vi "NotifyRegistered.vi"(2 "data string":string, 3 "ROS":T1={"topic port"=0, "Node"="", "topic"="", "type"="", "node port"=0, "error "={"status"=FALSE, "code"=0, "source"=""}, "Direction"=enum."Node", "APIs"=[], "Update (ms)"=1, "write queue"=1}) -> (1 "ROS out":T1={"topic port"=0, "Node"="", "topic"="", "type"="", "node port"=0, "error "={"status"=FALSE, "code"=0, "source"=""}, "Direction"=enum."Node", "APIs"=[], "Update (ms)"=1, "write queue"=1})   [LabVIEW 2012]
uses:
  <userlib>/ROSforLV/ROS/Code/SubVIs/_ROSControl.ctl
  <userlib>/ROSforLV/ROS/Code/SubVIs/_ROSDirection.ctl
panel:
  out "vi name":string
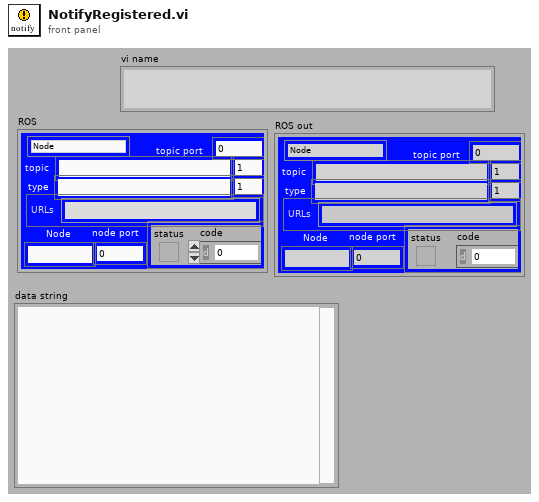
[diagram p1: front panel]
types:
  T1 = typedef "_ROSControl.ctl" = cluster{"topic port":u16, "Node":string, "topic":string, "type":string, "node port":u16, "error ":errorcluster, "Direction":T2, "APIs":string[], "Update (ms)":u16, "write queue":u16}
  T2 = typedef "_ROSDirection.ctl" = enum16{"Node", "Publisher", "Subscriber", "Service Client"}
  T3 = typedef "ServoInfo.ctl" = cluster{"vi name":string, "VI Refnum":refnum<vi>, "queue":refnum<queue>, "ROS":T1, "notifier":refnum<notifier>}
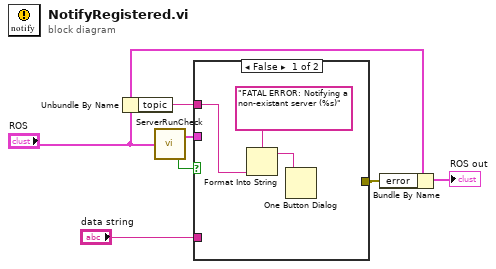
[diagram p0: block diagram]
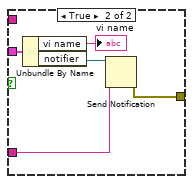
[diagram p2: hidden frame]
diagram:
  n1 = Unbundle By Name("ROS") -> ("topic"=w4:string)
  n2 = call <userlib>:"ServerRunCheck.vi"("ROS in"="ROS") -> ("Running?"=w5:bool, "ServerFound"=w6:T3)
  n3 = case shown="False" w5 {
    tunnel: "data string" -> [_ w15]
    tunnel: w6 -> [_ w14]
    tunnel: w4 -> [w8 _]
    tunnel: [_ w11] -> w2
    frame False {
      n4 = Format Into String(format string="FATAL ERROR: Notifying a non-existant server (%s)" ("message"), w8) -> (resulting string=w10:string)  [unwired: 2 in, 1 out]
      n5 = One Button Dialog(message=w10) -> ()  [unwired: 1 in, 1 out]
    }
    frame True {
      n6 = Unbundle By Name(w14) -> ("vi name"=→"vi name":string, "notifier"=w13:refnum<notifier>)
      n7 = Send Notification(notification=w15, notifier=w13) -> (error out=w11:errorcluster)  [unwired: 1 in, 1 out]
    }
  }
  n8 = Bundle By Name(cluster="ROS", "error"=w2) -> (→"ROS out":T1)
